vi "LVClass_Image ctor from subtraction.vi"(0 "Image (const)":refnum<class "Image.lvclass">, 5 "Image A":refnum<class "Image.lvclass">, 7 "Image B":refnum<class "Image.lvclass">, 11 "error in (no error)":errorcluster) -> (4 "Image (new)":refnum<class "Image.lvclass">, 6 "Image A (dup)":refnum<class "Image.lvclass">, 8 "Image B (dup)":refnum<class "Image.lvclass">, 15 "error out":errorcluster)   [LabVIEW 2020, in "Image.lvclass"]
doc: "Image constructor from a subtraction of two images : (new) image = imageA \\-\nimageB.\n\n--------------------------------------------------------------------------------\n\n<B>ImageIn </B> : Constant Pointer to Image object.\n<B>ImageOut </B> : Constant Pointer to Image object.\n<B>ImageA </B> : Image object.\n<B>ImageB </B> : Image object.\n<B>ErrorIn </B> : Error\n<B>ErrorOut </B> : Error\n\n--------------------------------------------------------------------------------"
uses:
  Image.lvclass
  Controls/Handle creation.ctl
  Image.lvclass/Image.ctl
  LVClass_Image read Image Compat ptr.vi
  LVClass_Image Read Image.vi
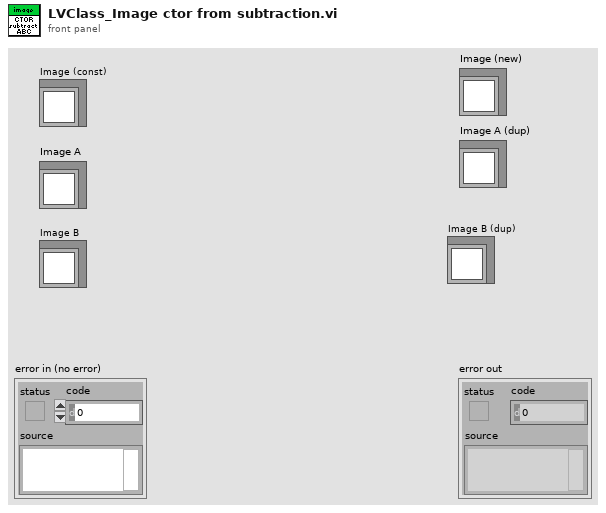
[diagram p1: front panel]
types:
  T1 = typedef "Handle creation.ctl" = enum16{"By ctor", "By write function"}
  T2 = typedef "ClassID.ctl" = i64
  T3 = typedef "Struct_Image.ctl" = cluster{"Image_Handler":T2, "Number of bits":T4, "ImageSize":T5}
  T4 = typedef "Data alignment enum.ctl" = enum16{"8", "16", "32"}
  T5 = typedef "Point2D.ctl" = cluster{"X":u32, "Y":u32}
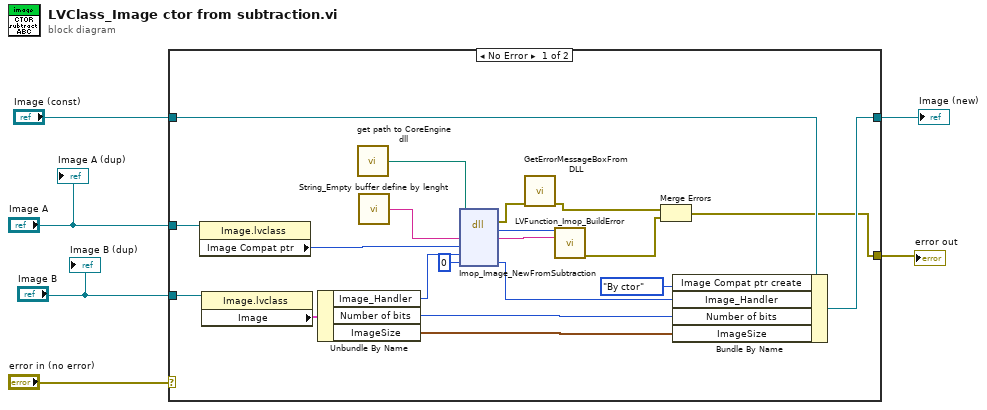
[diagram p0: block diagram]
diagram:
  n1 = case shown="No Error" "error in (no error)" {
    selector: "error in (no error)" -> [_ w28]
    tunnel: [w7 w28] -> w3
    tunnel: [w16 w27] -> w4
    tunnel: "Image (const)" -> [w17 w27]
    tunnel: "Image B" -> [w23 _]
    tunnel: "Image A" -> [w20 _]
    frame No Error {
      n2 = property class="Image.lvclass"(reference=w20) -> ("Image Compat ptr"=w19:T2)  [unwired: 1 in, 2 out]
      n3 = property class="Image.lvclass"(reference=w23) -> ("Image"=w14:T3)  [unwired: 1 in, 2 out]
      n4 = Unbundle By Name(w14) -> ("Image_Handler"=w13:T2, "Number of bits"=w12:T4, "ImageSize"=w11:T5)
      n5 = call "get path to CoreEngine dll.vi"() -> ("path to wavekit library"=w22:path)  [unwired: 14 in, 1 out]
      n6 = call "String_Empty buffer define by lenght.vi"() -> ("Empty buffer"=w26:string)  [unwired: 1 in]
      n7 = dll-call lib="D:/soft/HASO_v3/SVN_trunk/ImOpCoreEngine4_LV2011/DLLs/c_interface_vc100.dll" fn="Imop_Image_NewFromSubtraction"(path in=w22, "message"=w26, "Image 1"=w19, "Image 2"=w13, "Image3"=0) -> (error out=w21:errorcluster, "return type"=w25:i32, "message"=w24:string, "Image3"=w10:i64)  [unwired: 4 in, 1 out]
      n8 = call "GetErrorMessageBoxFromDLL.vi"("error IN"=w21) -> ("error OUT"=w9:errorcluster)  [unwired: 10 in]
      n9 = call "LVFunction_Imop_BuildError.vi"("code"=w25, "String to Prepend to source (\"\")"=w24) -> ("error out"=w8:errorcluster)  [unwired: 13 in]
      n10 = Merge Errors(w9, w8) -> (w7:errorcluster)
      n11 = Bundle By Name(cluster=w17, "Image Compat ptr create"=Handle_creation."By ctor", "Image_Handler"=w10, "Number of bits"=w12, "ImageSize"=w11) -> (w16:refnum<class "Image.lvclass">)
    }
    frame Error {
    }
  }
  "error out" <- w3
  "Image (new)" <- w4
  "Image A (dup)" <- "Image A"
  "Image B (dup)" <- "Image B"
